vi "test Copy Handle Data.vi"(8 "error in (no error)":errorcluster, 11 "TestCase in":refnum<class "Memory Manager Tests.lvclass">) -> (0 "error out":errorcluster, 3 "TestCase out":refnum<class "Memory Manager Tests.lvclass">)   [LabVIEW 2020, in "Memory Manager Tests.lvclass"]
uses:
  Memory Manager Tests.lvclass
  <vilib>/Utility/file.llb/Application Directory.vi
  <vilib>/Utility/libraryn.llb/Check if File or Folder Exists.vi
  <vilib>/addons/_JKI Toolkits/VI Tester/TestCase.llb/TestCase.lvclass
  C:/Program Files/National Instruments/LabVIEW 2024/vi.lib/addons/_JKI Toolkits/VI Tester/TestCase.llb/TestCase.lvclass
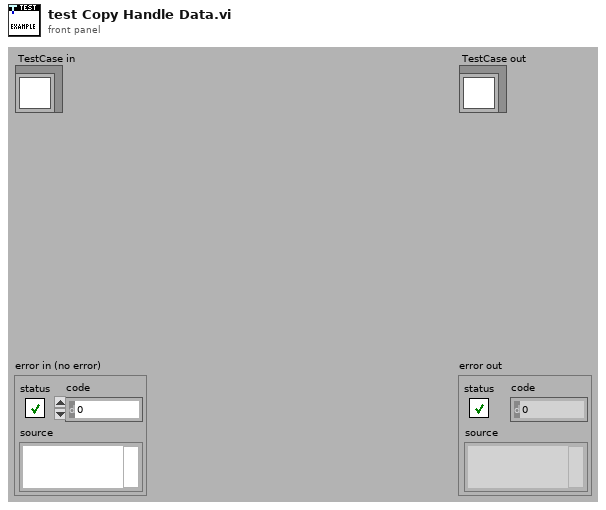
[diagram p1: front panel]
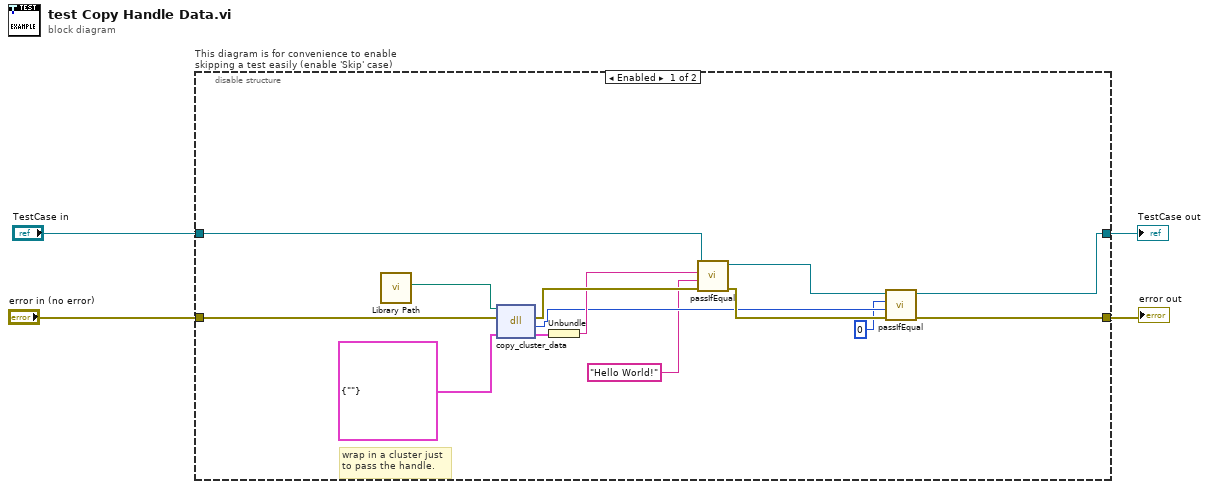
[diagram p0: block diagram]
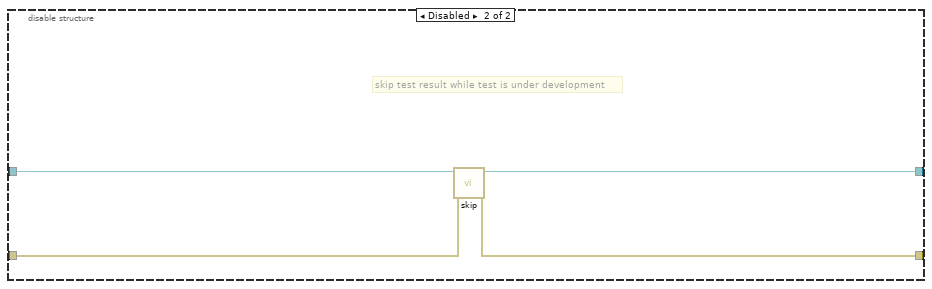
[diagram p2: hidden frame]
diagram:
  n1 = disable-structure "This diagram is for convenience to enable skipping a test easily (enable 'Skip' case)" shown="Enabled" {
    disable-tunnel: "TestCase in" -> [w18 w22]
    disable-tunnel: [w8 w20] -> w1
    disable-tunnel: [w10 w21] -> w3
    disable-tunnel: "error in (no error)" -> [w15 w19]
    frame Enabled {
      # "wrap in a cluster just\nto pass the handle."
      n2 = call "Library Path.vi"() -> ("Library Path"=w16:path)  [unwired: 11 in]
      n3 = dll-call lib="C:/Users/JamesMcNally/Documents/RustInterop/Rust-LabVIEW-Interop/target/debug/labview_test_library.dll" fn="copy_cluster_data"(path in=w16, error in=w15, "cluster"=cluster{string} {""}) -> (error out=w14:errorcluster, "return type"=w7:i32, "cluster"=w13:cluster{string})  [unwired: 1 in, 1 out]
      n4 = Unbundle(w13) -> (w12:string)
      n5 = call-dynamic "passIfEqual.vi"("error in (no error)"=w14, "y"="Hello World!", "x"=w12, "TestCase in"=w18) -> ("error out"=w17:errorcluster, "TestCase out"=w9:refnum<class "Memory Manager Tests.lvclass">)  [unwired: 6 in]
      n6 = call-dynamic "passIfEqual.vi"("error in (no error)"=w17, "y"=w7, "x"=0 ("return type"), "TestCase in"=w9) -> ("error out"=w10:errorcluster, "TestCase out"=w8:refnum<class "Memory Manager Tests.lvclass">)  [unwired: 6 in]
    }
    frame Disabled {
      # "skip test result while test is under development"
      n7 = call <vilib>:"skip.vi"("error in (no error)"=w19, "TestCase in"=w22) -> ("error out"=w21:errorcluster, "TestCase out"=w20:refnum<class "Memory Manager Tests.lvclass">)  [unwired: 8 in]
    }
  }
  "error out" <- w3
  "TestCase out" <- w1
